vi "Signed Min Max.vi"(3 "Min":dbl, 4 "Value":dbl, 5 "Max":dbl) -> (1 "Output":dbl)   [LabVIEW 2017]
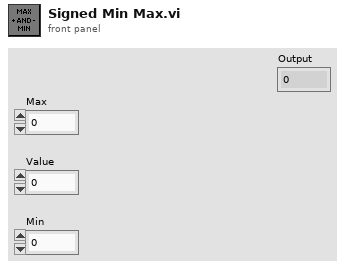
[diagram p1: front panel]
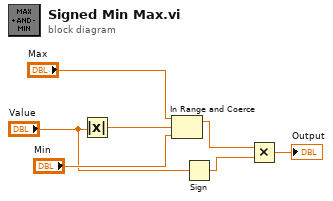
[diagram p0: block diagram]
diagram:
  n1 = Absolute Value(x="Value") -> (abs(x)=w7:dbl)
  n2 = In Range and Coerce(upper limit="Max", x=w7, lower limit="Min") -> (coerced(x)=w3:dbl)  [unwired: 1 out]
  n3 = Sign(1:"Value") -> (0:w2:dbl)
  n4 = Multiply(x=w3, y=w2) -> (x*y=→"Output":dbl)
